vi "2ndOrderDeltaSigma.vi"() -> ()   [LabVIEW 2014]
uses:
  <vilib>/Analysis/NI_AALBase.lvlib
panel:
  out "Bitstream":i32[](array[numeric])
  out "Bitstream":bool[](array[boolean])
  out "Delta Sigma Modulation":dbl[][](graph)
  out "SNR (dB)":dbl format="%#_4g"
  out "Sampled vs Continous Signal":dbl[][](graph)
  in  "Vref":dbl=1.5
  in  "Oversampling Factor":i32=8
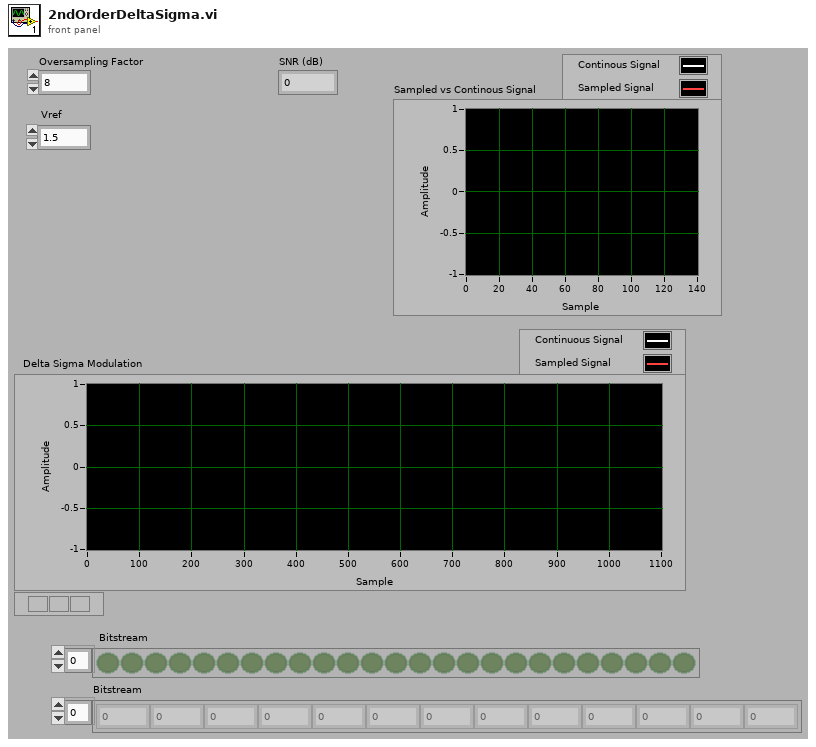
[diagram p1: front panel]
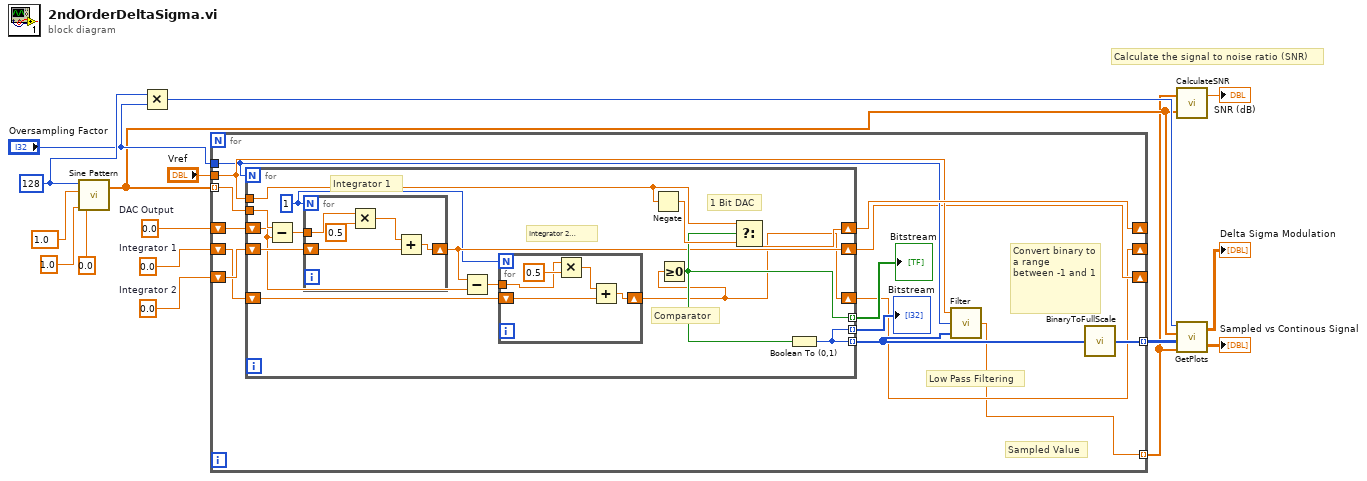
[diagram p0: block diagram]
diagram:
  w5 = 0.0  # Integrator 1
  w6 = 0.0  # Integrator 2
  w11 = 128 ("samples")
  w16 = 0.0  # DAC Output
  # "Calculate the signal to noise ratio (SNR)"
  n1 = call <vilib>:"Sine Pattern.vi"("cycles"=1.0, "phase(degrees)"=0.0, "amplitude"=1.0 ("phase(degrees)"), "samples"=w11) -> ("Sinusoidal Pattern"=w2:dbl[])  [unwired: 1 out]
  n2 = Multiply(x=w11, y="Oversampling Factor") -> (x*y=w7:i32)
  n3 = for {
    shift-right: [w29] -> _
    shift-left: w16 -> [w30]
    tunnel: "Vref" -> [w25]
    tunnel: "Oversampling Factor" -> [w24]
    tunnel: w2 -> [w28] mode=indexing
    tunnel: [w26] -> w8 mode=indexing
    tunnel: [w17] -> w1 mode=indexing
    shift-right: [w20] -> _
    shift-left: w6 -> [w21]
    shift-right: [w18] -> _
    shift-left: w5 -> [w19]
    # "Sampled Value"
    # "Low Pass Filtering"
    # "Convert binary to a range\nbetween -1 and 1"
    n4 = for {
      N: w24 -> [_]
      tunnel: w28 -> [w44]
      shift-right: [w41] -> w29
      shift-left: w30 -> [w32]
      tunnel: w25 -> [w42]
      tunnel: [w40] -> w27 mode=indexing
      tunnel: [w39] -> w23 mode=indexing
      tunnel: [w40] -> w22 mode=indexing
      shift-right: [w36] -> w20
      shift-left: w21 -> [w37]
      shift-right: [w31] -> w18
      shift-left: w19 -> [w33]
      w34 = 1
      # "Integrator 2 Integrator 2"
      # "Integrator 1"
      # "1 Bit DAC"
      # "Comparator"
      n5 = Subtract(x=w44, y=w32) -> (x-y=w38:dbl)
      n6 = for {
        N: w34 -> [_]
        tunnel: w38 -> [w51]
        shift-right: [w53] -> w36
        shift-left: w37 -> [w54]
        n7 = Multiply(x=w51, y=0.5) -> (x*y=w52:dbl)
        n8 = Add(x=w52, y=w54) -> (x+y=w53:dbl)
      }
      n9 = Subtract(x=w36, y=w32) -> (x-y=w35:dbl)
      n10 = for {
        N: w34 -> [_]
        shift-right: [w48] -> w31
        shift-left: w33 -> [w49]
        tunnel: w35 -> [w45]
        n11 = Multiply(x=w45, y=0.5) -> (x*y=w46:dbl)
        n12 = Add(x=w46, y=w49) -> (x+y=w48:dbl)
      }
      n13 = Negate(x=w42) -> (-x=w43:dbl)
      n14 = Greater Or Equal To 0?(x=w31) -> (x >= 0?=w39:bool)
      n15 = Select(t=w42, s=w39, f=w43) -> (s? t:f=w41:dbl)
      n16 = Boolean To (0,1)(Boolean=w39) -> (0, 1=w40:i16)
    }
    "Bitstream" <- w23
    "Bitstream" <- w22
    n17 = call "Filter.vi"("Bits"=w27, "Oversampling Factor"=w24, "Vref"=w25) -> ("Sample"=w17:dbl)
    n18 = call "BinaryToFullScale.vi"("Array 2"=w27) -> ("Array"=w26:i16[])
  }
  n19 = call "CalculateSNR.vi"("Original Signal"=w2, "Sampled Signal"=w1) -> ("SNR"=→"SNR (dB)":dbl)  [unwired: 1 in]
  n20 = call "GetPlots.vi"("Sampled Signal"=w1, "Two Level Signal"=w8, "Sinusoidal Pattern"=w2, "No. of Oversamples"=w7) -> ("Sampled vs Continuous Signal"=→"Sampled vs Continous Signal":dbl[][], "Delta Sigma Modulation Signal"=→"Delta Sigma Modulation":dbl[][])
